vi "Get Configuration Metadata.vi"(8 "error in (no error)":errorcluster, 11 "MeasurementPluginService in":refnum<class "MeasurementPluginService.lvclass">) -> (0 "error out":errorcluster, 3 "Metadata Value":T2(array[cluster]))   [LabVIEW 2020, in "MeasurementLink Measurement Server.lvlib"]
uses:
  MeasurementLink Measurement Server.lvlib
  TypeDefs/ConfigurationParameter_AnnotationsEntry.ctl
  Classes/MeasurementPluginService/MeasurementPluginService.lvclass
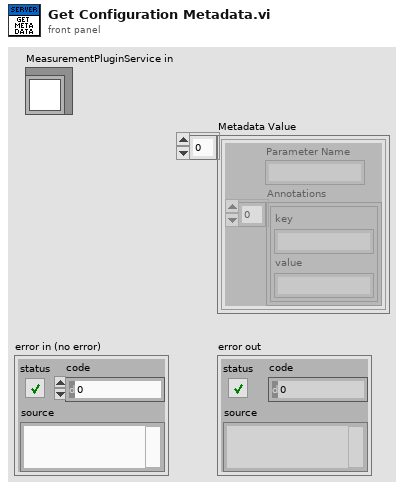
[diagram p1: front panel]
types:
  T1 = typedef "MeasurementLink Measurement Server.lvlib/ConfigurationParameter_AnnotationsEntry.ctl" = cluster{"key":string, "value":string}
  T2 = cluster{"Parameter Name":string, "Annotations":T1[]}[]
  T3 = typedef "MeasurementLink Measurement Server.lvlib/MeasurementPluginService.lvclass/Plugin Paths.ctl" = cluster{"Get Measurement Details VI Path":path, "Get Type Specializations VI Path":path, "Get UI Details VI Path":path, "Measurement Logic VI Path":path, "Measurement Configuration CTL Path":path, "Measurement Results CTL Path":path}
  T4 = typedef "MeasurementLink Measurement Server.lvlib/Parameter Type Specialization.ctl" = cluster{"Parameter Name":string, "Type Specialization":T5, "Annotations":cluster{"Key":T6, "Value":string}[]}
  T5 = typedef "MeasurementLink Measurement Server.lvlib/Type Specialization.ctl" = enum16{"none", "pin", "path", "enum"}
  T6 = typedef "MeasurementLink Measurement Server.lvlib/Type Specialization Key.ctl" = enum16{"none", "pin.instrument_type", "enum.values"}
  T7 = cluster{"Parameter Name":string, "Annotations":T1[]}
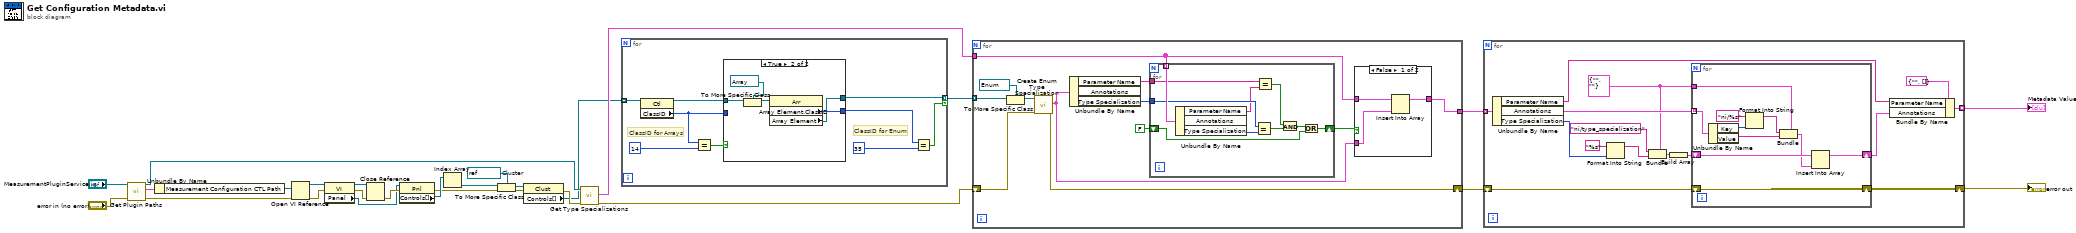
[diagram p0: block diagram]
diagram:
  w17 = refnum<vi> refnum  # Cluster
  n1 = call-dynamic "Get Plugin Paths.vi"("error in (no error)"="error in (no error)", "MeasurementPluginService in"="MeasurementPluginService in") -> ("error out"=w6:errorcluster, "Plugin Paths"=w13:T3, "MeasurementPluginService out"=w3:refnum<class "MeasurementPluginService.lvclass">)  [unwired: 7 in]
  n2 = Unbundle By Name(w13) -> ("Measurement Configuration CTL Path"=w8:path)
  n3 = Open VI Reference(vi path=w8, error in (no error)=w6) -> (vi reference=w7:refnum<vi>, error out=w19:errorcluster)  [unwired: 4 in]
  n4 = property class="VI"(reference=w7, error in=w19) -> (reference out=w12:refnum<vi>, error out=w10:errorcluster, "Panel"=w9:refnum<vi>)
  n5 = Close Reference(reference=w12, error in (no error)=w10) -> (error out=w11:errorcluster)
  n6 = property class="Pnl"(reference=w9, error in=w11) -> (error out=w16:errorcluster, "Controls[]"=w20:refnum<vi>[])  [unwired: 1 out]
  n7 = Index Array(array=w20) -> (element=w18:refnum<vi>)  [unwired: 1 in]
  n8 = To More Specific Class(target class=w17, reference=w18, error in=w16) -> (specific class reference=w15:refnum<vi>, error out=w5:errorcluster)
  n9 = property class="Clust"(reference=w15, error in=w5) -> (error out=w4:errorcluster, "Controls[]"=w1:refnum<vi>[])  [unwired: 1 out]
  n10 = call-dynamic "Get Type Specializations.vi"("error in (no error)"=w4, "MeasurementPluginService in"=w3) -> ("error out"=w24:errorcluster, "Type Specializations"=w22:T4[])  [unwired: 7 in, 1 out]
  n11 = for {
    tunnel: w1 -> [w36] mode=indexing
    tunnel: [w33] -> w23 mode=indexing if=w28
    # "ClassID for Enum"
    # "ClassID for Arrays"
    n12 = property class="Ctl"(reference=w36) -> (reference out=w34:refnum<vi>, "ClassID"=w32:u32)  [unwired: 1 in, 1 out]
    n13 = Equal?(x=w32, y=u32 14) -> (x = y?=w31:bool)
    n14 = case shown="True" w31 {
      tunnel: w34 -> [w37 w43]
      tunnel: [w37 w39] -> w33
      tunnel: [w38 w41] -> w29
      tunnel: w32 -> [w38 _]
      frame False {
      }
      frame True {
        n15 = To More Specific Class(target class=refnum<vi> refnum ("Enum reference in"), reference=w43) -> (specific class reference=w42:refnum<vi>)  [unwired: 1 in, 1 out]
        n16 = property class="Arr"(reference=w42) -> ("Array Element.ClassID"=w41:u32, "Array Element"=w39:refnum<vi>)  [unwired: 1 in, 2 out]
      }
    }
    n17 = Equal?(x=w29, y=u32 35) -> (x = y?=w28:bool)
  }
  n18 = for {
    shift-right: [w53] -> w25
    shift-left: w24 -> [w54]
    tunnel: w23 -> [w51] mode=indexing
    tunnel: w22 -> [w44]
    tunnel: [w45] -> w21
    n19 = To More Specific Class(target class=refnum<vi> refnum ("Enum reference in"), reference=w51) -> (specific class reference=w55:refnum<vi>)  [unwired: 1 in, 1 out]
    n20 = call "Create Enum Type Specialization.vi"("error in (no error)"=w54, "Enum reference in"=w55) -> ("error out"=w53:errorcluster, "Parameter Type Specialization Output"=w46:T4)  [unwired: 6 in, 1 out]
    n21 = Unbundle By Name(w46) -> ("Parameter Name"=w50:string, "Type Specialization"=w49:T5)  [unwired: 1 out]
    n22 = for {
      tunnel: w44 -> [w69] mode=indexing
      tunnel: w50 -> [w66]
      tunnel: w49 -> [w67]
      shift-right: [w62] -> w47
      shift-left: FALSE -> [w60]
      n23 = Unbundle By Name(w69) -> ("Parameter Name"=w65:string, "Type Specialization"=w68:T5)  [unwired: 1 out]
      n24 = Equal?(x=w67, y=w68) -> (x = y?=w63:bool)
      n25 = Equal?(x=w66, y=w65) -> (x = y?=w64:bool)
      n26 = And(x=w64, y=w63) -> (x .and. y?=w61:bool)
      n27 = Or(x=w61, y=w60) -> (x .or. y?=w62:bool)
    }
    n28 = case shown="False" w47 {
      tunnel: w44 -> [w58 w59]
      tunnel: w46 -> [w57 _]
      tunnel: [w56 w59] -> w45
      frame False {
        n29 = Insert Into Array(array=w58, new element=w57) -> (w56:T4[])  [unwired: 1 in]
      }
      frame True {
      }
    }
  }
  n30 = for {
    tunnel: w21 -> [w84] mode=indexing
    shift-right: [w80] -> w26
    shift-left: w25 -> [w81]
    tunnel: [w82] -> w27 mode=indexing
    w71 = T1 {"key"="", "value"=""} ("ConfigurationParameter_AnnotationsEntry")
    n31 = Unbundle By Name(w84) -> ("Parameter Name"=w70:string, "Annotations"=w75:cluster{"Key":T6, "Value":string}[], "Type Specialization"=w79:T5)
    n32 = Format Into String(format string="%s", w79) -> (resulting string=w77:string)  [unwired: 2 in, 1 out]
    n33 = Bundle(cluster=w71, "key"="ni/type_specialization" ("Value"), "value"=w77) -> (w72:T1)
    n34 = Build Array(w72) -> (w73:T1[])
    n35 = for {
      shift-right: [w94] -> w80
      shift-left: w81 -> [w94]
      tunnel: w75 -> [w93] mode=indexing
      shift-right: [w86] -> w74
      shift-left: w73 -> [w88]
      tunnel: w71 -> [w85]
      n36 = Unbundle By Name(w93) -> ("Key"=w91:T6, "Value"=w89:string)
      n37 = Format Into String(format string="ni/%s", w91) -> (resulting string=w90:string)  [unwired: 2 in, 1 out]
      n38 = Bundle(cluster=w85, "key"=w90, "value"=w89) -> (w87:T1)
      n39 = Insert Into Array(array=w88, new element=w87) -> (w86:T1[])  [unwired: 1 in]
    }
    n40 = Bundle By Name(cluster=T7 {"Parameter Name"="", "Annotations"=[]} ("Cluster"), "Parameter Name"=w70, "Annotations"=w74) -> (w82:T7)
  }
  "error out" <- w26
  "Metadata Value" <- w27
